vi "Drop Event into subVI.vi"(10 "VI":refnum<class "VI.lvclass">, 11 "Project":refnum<class "Project.lvclass">) -> (0 "error out":errorcluster)   [LabVIEW 2020, in "Panther Dashboard.lvlib"]
uses:
  Panther Dashboard.lvlib
  Class/Project/Project.lvclass
  Class/VI/VI.lvclass
  C:/GitClones/PantherDashboard/src/LabVIEW/Panther Dashboard/Class/LabVIEWItem/LabVIEWItem.lvclass
  Class/Project/Project.lvclass/Project.ctl
  Class/LabVIEWItem/LabVIEWItem.lvclass/LabVIEWItem.ctl
  Class/LabVIEWItem/Read Item Name.vi
  Class/LabVIEWItem/Read Item Path.vi
  Class/Project/Read Main App Inst Ref.vi
  Class/Project/Read Target Ref.vi
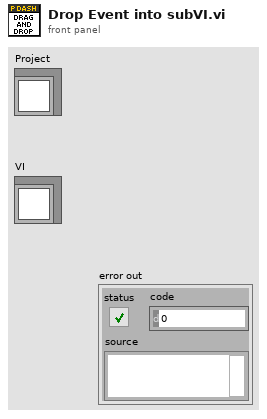
[diagram p1: front panel]
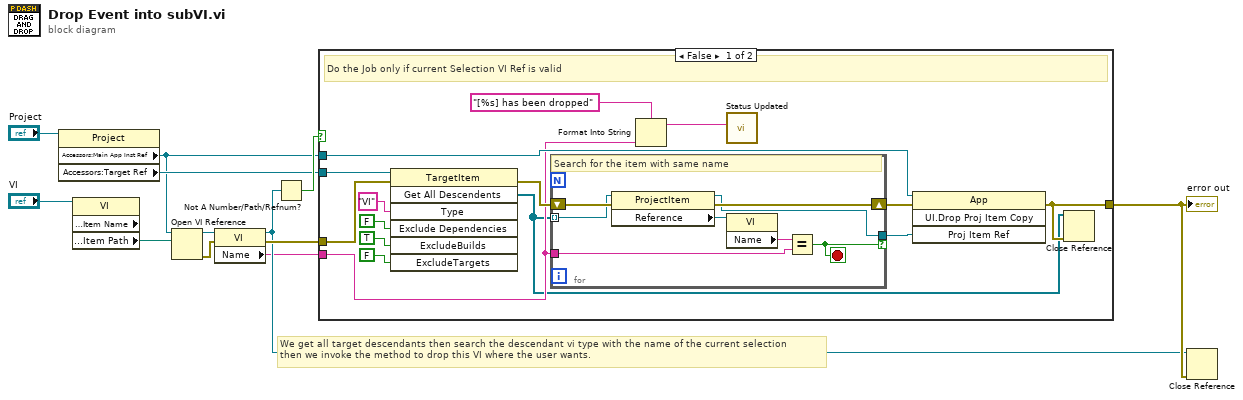
[diagram p0: block diagram]
diagram:
  # "We get all target descendants then search the descendant vi type with the name of the current selection\nthen we invoke the method to drop this VI where the user wants."
  n1 = property class="Project"(reference="Project") -> ("Accessors:Main App Inst Ref"=w7:refnum<vi>, "Accessors:Target Ref"=w8:refnum<vi>)  [unwired: 1 in, 2 out]
  n2 = property class="VI" props=["Accessors:Item Name", "Accessors:Item Path"](reference="VI") -> ("Accessors:Item Path"=w10:path)  [unwired: 1 in, 3 out]
  n3 = Open VI Reference(application reference (local)=w7, vi path=w10) -> (vi reference=w3:refnum<vi>, error out=w5:errorcluster)  [unwired: 4 in]
  n4 = property class="VI"(reference=w3, error in=w5) -> (reference out=w2:refnum<vi>, error out=w4:errorcluster, "Name"=w1:string)
  n5 = Not A Number/Path/Refnum?(number/path/refnum=w2) -> (NaN/Path/Refnum?=w12:bool)
  n6 = case shown="False" w12 {
    tunnel: [w14 _] -> w6
    tunnel: w8 -> [w20 _]
    tunnel: w7 -> [w18 _]
    tunnel: w1 -> [w15 _]
    tunnel: w4 -> [w27 _]
    frame False {
      # "Do the Job only if current Selection VI Ref is valid"
      n7 = invoke class="TargetItem" method="Get All Descendents"(reference=w20, error in=w27, "Type"="VI", "Exclude Dependencies"=FALSE ("ExcludeDependencies"), "ExcludeBuilds"=TRUE, "ExcludeTargets"=FALSE) -> (error out=w26:errorcluster, "All Descendents"=w13:refnum<vi>[])  [unwired: 1 in, 5 out]
      n8 = for {
        tunnel: w13 -> [w32] mode=indexing
        tunnel: [w31] -> w19 if=w33
        tunnel: w15 -> [w29]
        shift-right: [w34] -> w25
        shift-left: w26 -> [w35]
        stop <- w33 stop-if-true
        # "Search for the item with same name"
        n9 = property class="ProjectItem"(reference=w32, error in=w35) -> (reference out=w31:refnum<vi>, error out=w34:errorcluster, "Reference"=w30:refnum<vi>)
        n10 = property class="VI"(reference=w30) -> ("Name"=w28:string)  [unwired: 1 in, 2 out]
        n11 = Equal?(x=w28, y=w29) -> (x = y?=w33:bool)
      }
      n12 = Format Into String(format string="[%s] has been dropped", w15) -> (resulting string=w17:string)  [unwired: 2 in, 1 out]
      n13 = call "Status Updated.vi"("Status"=w17) -> ()  [unwired: 10 in, 1 out]
      n14 = invoke class="App" method="UI.Drop Proj Item Copy"(reference=w18, error in=w25, "Proj Item Ref"=w19) -> (error out=w14:errorcluster)  [unwired: 1 in, 3 out]
      n15 = Close Reference(reference=w13, error in (no error)=w14) -> ()  [unwired: 1 out]
    }
    frame True {
    }
  }
  "error out" <- w6
  n16 = Close Reference(reference=w2, error in (no error)=w6) -> ()  [unwired: 1 out]
